vi "Async.Engine.Write Data to HW.vi"(8 "error in":errorcluster, 11 "Async in":refnum<class "VS Inline Async API (Express).lvclass">) -> (0 "error out":errorcluster, 3 "Async out":refnum<class "VS Inline Async API (Express).lvclass">)   [LabVIEW 2027, in "VS Inline Async API (Express).lvlib" / "VS Inline Async API (Express).lvclass"]
uses:
  VS Inline Async API (Express).lvclass
  VS Inline Async API (Express).lvclass/VS Inline Async API (Express).ctl
  _Data Access Engine (Express)/Data Access Engine (Express)/Data Access Engine (Express).lvclass/Data Access Engine (Express).ctl
  _Data Access Engine (Express)/Access Type Classes/Read/Read.lvclass/Read.ctl
  _Data Access Engine (Express)/Access Type Classes/Read/Read.EngineData.vi
  <userlib>/Custom Device Interfaces_v1.lvlibp/CustomDeviceAPI/Custom Device API.lvclass
  _Data Access Engine (Express)/Data Access Engine (Express)/Data Access Engine (Express).lvclass
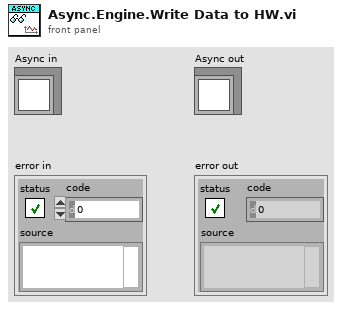
[diagram p1: front panel]
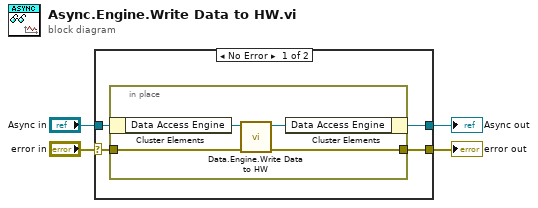
[diagram p0: block diagram]
diagram:
  n1 = case shown="No Error" "error in" {
    selector: "error in" -> [w6 w14]
    tunnel: [w5 w14] -> w3
    tunnel: [w7 w13] -> w1
    tunnel: "Async in" -> [w8 w13]
    frame No Error {
      n2 = in-place {
        in-place-border: w6 -> [w12]
        in-place-border: [w9] -> w5
        n3 = in-place-cluster #1(w8) -> ("Data Access Engine"=w11:refnum<class "Data Access Engine (Express).lvclass">)
        n4 = call "Data.Engine.Write Data to HW.vi"("error in"=w12, "Data Access API in"=w11) -> ("error out"=w9:errorcluster, "Data Access API out"=w10:refnum<class "Data Access Engine (Express).lvclass">)  [unwired: 8 in]
        n5 = in-place-cluster #1("Data Access Engine"=w10) -> (w7:refnum<class "VS Inline Async API (Express).lvclass">)
      }
    }
    frame Error {
    }
  }
  "error out" <- w3
  "Async out" <- w1
